vi "changeState.vi"(8 "error in (no error)":errorcluster, 10 "State:":T1, 11 "Model in":refnum<class "Model.lvclass">) -> (0 "error out":errorcluster, 3 "Model out":refnum<class "Model.lvclass">)   [LabVIEW 2013, in "Model.lvclass"]
uses:
  Model.lvclass
  Typedefs/StateSelector.ctl
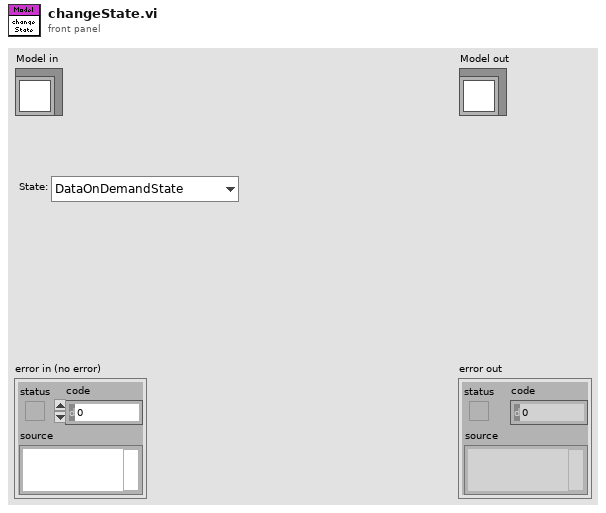
[diagram p1: front panel]
types:
  T1 = typedef "StateSelector.ctl" = enum16{"DataOnDemandState", "DataStreamingState", "FaultState", "OffState", "StandbyState"}
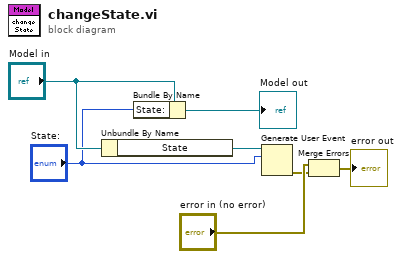
[diagram p0: block diagram]
diagram:
  n1 = Unbundle By Name("Model in") -> ("State"=w7:refnum<user-event>)
  n2 = Bundle By Name(cluster="Model in", "State:"="State:") -> (→"Model out":refnum<class "Model.lvclass">)
  n3 = Generate User Event(user event=w7, event data cluster="State:") -> (error out=w3:errorcluster)  [unwired: 2 in, 1 out]
  n4 = Merge Errors("error in (no error)", w3) -> (→"error out":errorcluster)
